vi "StringArray TO step.vi"(10 "ItemNames":string[](array[string])) -> (2 "STEP":T1 {"Tempo Step[s]" format="%#.1f"})   [LabVIEW 2019]
uses:
  controls/STEP.ctl
  controls/Caratteristiche step.ctl
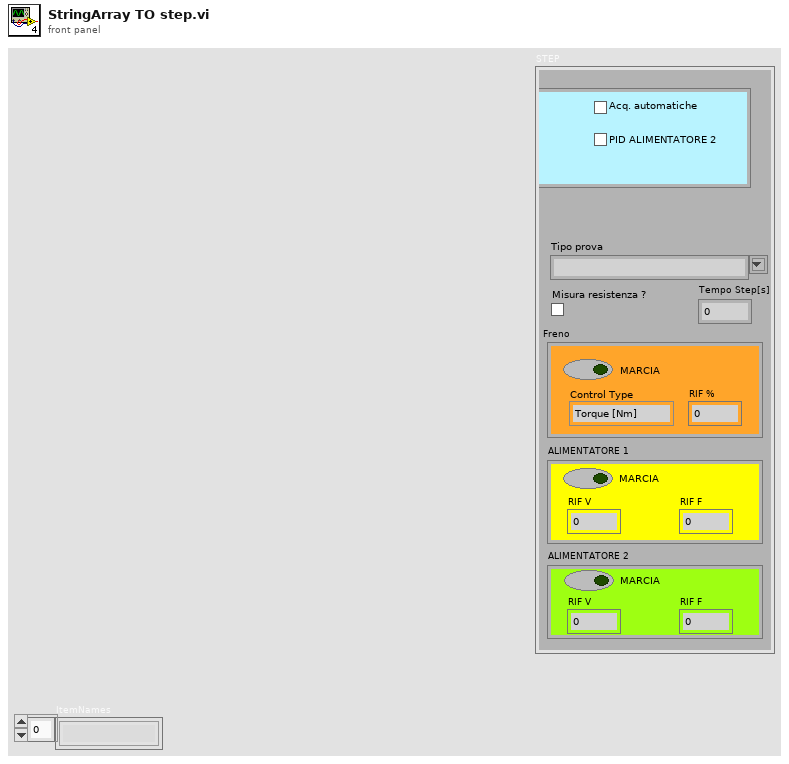
[diagram p1: front panel]
types:
  T1 = typedef "STEP.ctl" = cluster{"Tipo prova":string, "Misura resistenza ?":bool, "Tempo Step[s]":dbl, "Freno":cluster{"MARCIA":bool, "Control Type":enum32{"Torque [Nm]", "Power [W]", "Speed [RPM]", "Corrente [A]"}, "RIF %":dbl}, "ALIMENTATORE 1":cluster{"MARCIA":bool, "RIF V":dbl, "RIF F":dbl}, "ALIMENTATORE 2":cluster{"MARCIA":bool, "RIF V":dbl, "RIF F":dbl}, "Caratteristiche step":T2}
  T2 = typedef "Caratteristiche step.ctl" = cluster{"Attendi stabilizz.":bool, "Acq. fine step?":bool, "Acq. automatiche":bool, "PID FRENO":bool, "PID ALIMENTATORE 1":bool, "PID ALIMENTATORE 2":bool, "CAMBIA PROVA SE EQ. TERMICO":bool}
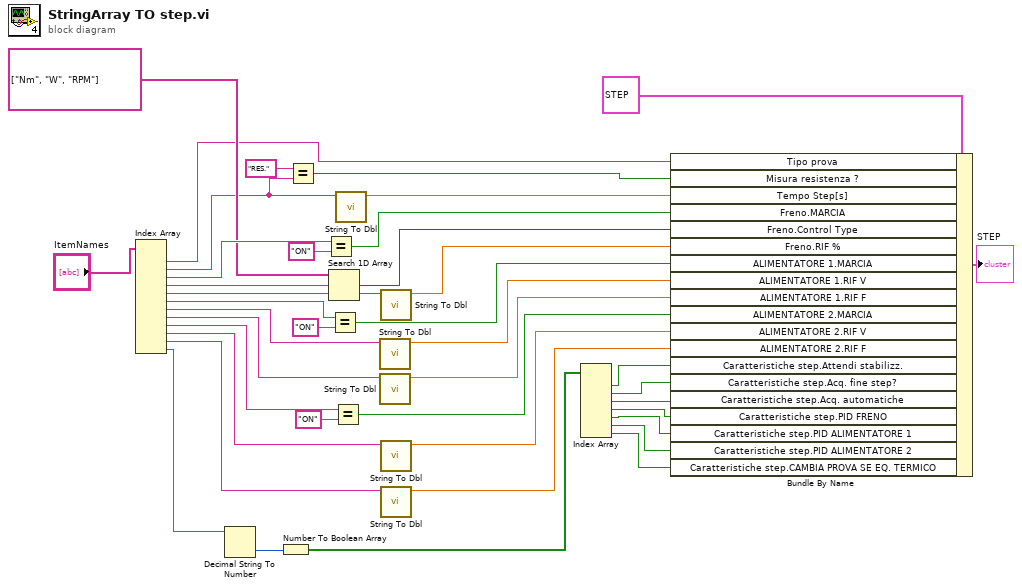
[diagram p0: block diagram]
diagram:
  n1 = Index Array(array="ItemNames") -> (element #1=w11:string, element #2=w14:string, element #3=w37:string, element #4=w33:string, element #5=w31:string, element #6=w28:string, element #7=w26:string, element #8=w24:string, element #9=w21:string, element #10=w19:string, element #11=w18:string, element #12=w10:string)  [unwired: 12 in]
  n2 = Decimal String To Number(string=w10) -> (number=w9:i32)  [unwired: 2 in, 1 out]
  n3 = Number To Boolean Array(number=w9) -> (Boolean array=w8:bool[])
  n4 = Equal?(x="RES.", y=w14) -> (x = y?=w12:bool)
  n5 = Equal?(x=w37, y="ON") -> (x = y?=w35:bool)
  n6 = Search 1D Array(1D array=string[] ["Nm", "W", "RPM"], element=w33) -> (index of element=w32:i32)  [unwired: 1 in]
  n7 = Equal?(x=w28, y="ON") -> (x = y?=w27:bool)
  n8 = Equal?(x=w21, y="ON") -> (x = y?=w20:bool)
  n9 = call "String To Dbl.vi"("String"=w14) -> ("Numeric"=w38:dbl)  [unwired: 10 in]
  n10 = call "String To Dbl.vi"("String"=w26) -> ("Numeric"=w25:dbl)  [unwired: 10 in]
  n11 = call "String To Dbl.vi"("String"=w24) -> ("Numeric"=w23:dbl)  [unwired: 10 in]
  n12 = call "String To Dbl.vi"("String"=w31) -> ("Numeric"=w30:dbl)  [unwired: 10 in]
  n13 = call "String To Dbl.vi"("String"=w19) -> ("Numeric"=w17:dbl)  [unwired: 10 in]
  n14 = call "String To Dbl.vi"("String"=w18) -> ("Numeric"=w16:dbl)  [unwired: 10 in]
  n15 = Index Array(array=w8) -> (element #1=w7:bool, element #2=w6:bool, element #3=w5:bool, element #4=w4:bool, element #5=w3:bool, element #6=w2:bool, element #7=w1:bool)  [unwired: 7 in]
  n16 = Bundle By Name(cluster=T1 {"Tipo prova"="", "Misura resistenza ?"=FALSE, "Tempo Step[s]"=0.0, "Freno"={"MARCIA"=FALSE, "Control Type"=enum."Torque [Nm]", "RIF %"=0.0}, "ALIMENTATORE 1"={"MARCIA"=FALSE, "RIF V"=0.0, "RIF F"=0.0}, "ALIMENTATORE 2"={"MARCIA"=FALSE, "RIF V"=0.0, "RIF F"=0.0}, "Caratteristiche step"={"Attendi stabilizz."=FALSE, "Acq. fine step?"=FALSE, "Acq. automatiche"=FALSE, "PID FRENO"=FALSE, "PID ALIMENTATORE 1"=FALSE, "PID ALIMENTATORE 2"=FALSE, "CAMBIA PROVA SE EQ. TERMICO"=FALSE}} ("MODIFICA STEP"), "Tipo prova"=w11, "Misura resistenza ?"=w12, "Tempo Step[s]"=w38, "Freno.MARCIA"=w35, "Freno.Control Type"=w32, "Freno.RIF %"=w30, "ALIMENTATORE 1.MARCIA"=w27, "ALIMENTATORE 1.RIF V"=w25, "ALIMENTATORE 1.RIF F"=w23, "ALIMENTATORE 2.MARCIA"=w20, "ALIMENTATORE 2.RIF V"=w17, "ALIMENTATORE 2.RIF F"=w16, "Caratteristiche step.Attendi stabilizz."=w7, "Caratteristiche step.Acq. fine step?"=w6, "Caratteristiche step.Acq. automatiche"=w5, "Caratteristiche step.PID FRENO"=w4, "Caratteristiche step.PID ALIMENTATORE 1"=w3, "Caratteristiche step.PID ALIMENTATORE 2"=w2, "Caratteristiche step.CAMBIA PROVA SE EQ. TERMICO"=w1) -> (→"STEP":T1)
